vi "Read Pulse Configuration.vi"(8 "error in (no error)":errorcluster, 11 "DAQmx Synthesizer in":refnum<class "DAQmx Synthesizer.lvclass">) -> (0 "error out":errorcluster, 2 "Configuration":T1={"Pre-trigger duration"=0.01, "Post-trigger duration"=0.1, "Rate"=1000000.0, "Ranges"=[10.0], "Re-name channels"=[], "Active channels"="0:1", "External clock"=FALSE} {"Rate" format="%#_8pHz"; "Post-trigger duration" format="%#_6ps"; "Pre-trigger duration" format="%#_6ps"; "Ranges" format="%#_6pV"}, 3 "DAQmx Synthesizer out":refnum<class "DAQmx Synthesizer.lvclass">)   [LabVIEW 2019, in "DAQmx Synthesizer.lvclass"]
uses:
  DAQmx Synthesizer.lvclass
  Instruments/Pulse Driver/Pusle Driver Configuration.ctl
  DAQmx Synthesizer.lvclass/DAQmx Synthesizer.ctl
  <vilib>/Waveform/WDTOps.llb/WDT Waveform Duration DBL.vi
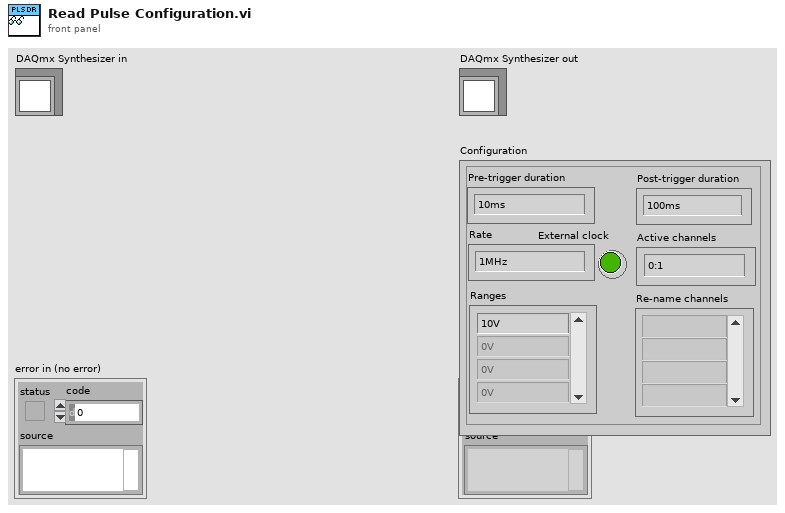
[diagram p1: front panel]
types:
  T1 = typedef "Pusle Driver Configuration.ctl" = cluster{"Pre-trigger duration":dbl, "Post-trigger duration":dbl, "Rate":dbl, "Ranges":dbl[], "Re-name channels":string[], "Active channels":string, "External clock":bool}
  T2 = typedef "DAQmx Synthesizer Configuration.ctl" = cluster{"Ranges":dbl[], "Channel names":string[], "Output channels":string, "File Path Control":path}
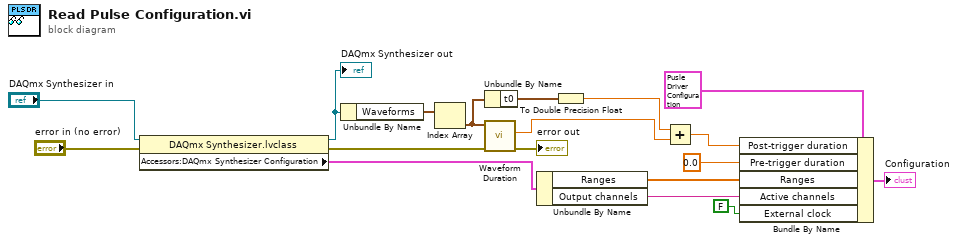
[diagram p0: block diagram]
diagram:
  n1 = property class="DAQmx Synthesizer.lvclass"(reference="DAQmx Synthesizer in", error in="error in (no error)") -> (reference out=w9:refnum<class "DAQmx Synthesizer.lvclass">, error out=w2:errorcluster, "Accessors:DAQmx Synthesizer Configuration"=w14:T2)
  "DAQmx Synthesizer out" <- w9
  n2 = Unbundle By Name(w9) -> ("Waveforms"=w8:waveform(dbl)[])
  n3 = Index Array(array=w8) -> (element=w7:waveform(dbl))  [unwired: 1 in]
  n4 = Unbundle By Name(w7) -> ("t0"=w6:timestamp)
  n5 = call-poly <vilib>:"Waveform Duration.vi"("error in (no error)"=w2, "waveform in"=w7) -> ("error out"=→"error out":errorcluster, "duration"=w4:dbl)  [unwired: 7 in, 1 out]
  n6 = Unbundle By Name(w14) -> ("Ranges"=w12:dbl[], "Output channels"=w11:string)
  n7 = To Double Precision Float(number=w6) -> (double precision float=w5:dbl)
  n8 = Add(x=w5, y=w4) -> (x+y=w3:dbl)
  n9 = Bundle By Name(cluster=T1 {"Pre-trigger duration"=0.01, "Post-trigger duration"=0.1, "Rate"=1000000.0, "Ranges"=[10.0], "Re-name channels"=[], "Active channels"="0:1", "External clock"=FALSE} ("Configuration"), "Post-trigger duration"=w3, "Pre-trigger duration"=0.0, "Ranges"=w12, "Active channels"=w11, "External clock"=FALSE) -> (→"Configuration":T1)
